vi "RT Driver_Get Date And Time NTP V4.vi"(8 "error in (no error) 2":errorcluster, 10 "port or service name":u16=123, 11 "Timer Server IP Address":string="206.246.122.250") -> (0 "error out":errorcluster, 1 "Last error":errorcluster, 2 "Server Reached":bool, 3 "Server Time (Transmit TimeStamp)":timestamp format="%<%.6X\n%x>T", 5 "Offset (s)":dbl format="%_4p")   [LabVIEW 2013, in "SNTP Light Custom Device Engine.lvlib"]
uses:
  SNTP Light Custom Device Engine.lvlib
panel:
  out "x+y 2":dbl format="%.6f"
  out "x+y":dbl format="%.6f"
  out "Server Time (Receive TimeStamp)":timestamp format="%<%.6X\n%x>T"
  out "Round Trip Delay (s)":dbl
  out "current time":timestamp format="%<%.6X\n%x>T"
  out "Local Time (Destination TimeStamp)":timestamp format="%<%.6X\n%x>T"
  # "64.90.182.55"
  # "129.6.15.28"
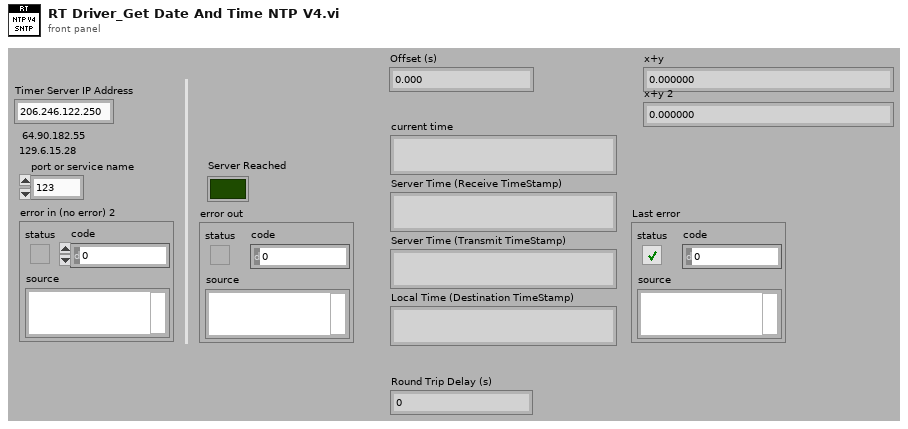
[diagram p1: front panel]
types:
  T1 = cluster{"LI|VN|Mode":u8, "Stratum":u8, "Poll":u8, "Precision":u8, "Root Delay":u32, "Root Dispersion":u32, "Reference Identifier":u32, "Reference Timestamp":fxp<+,64,32>, "Originate Timestamp":fxp<+,64,32>, "Receive Timestamp":fxp<+,64,32>, "Transmit Timestamp":fxp<+,64,32>}
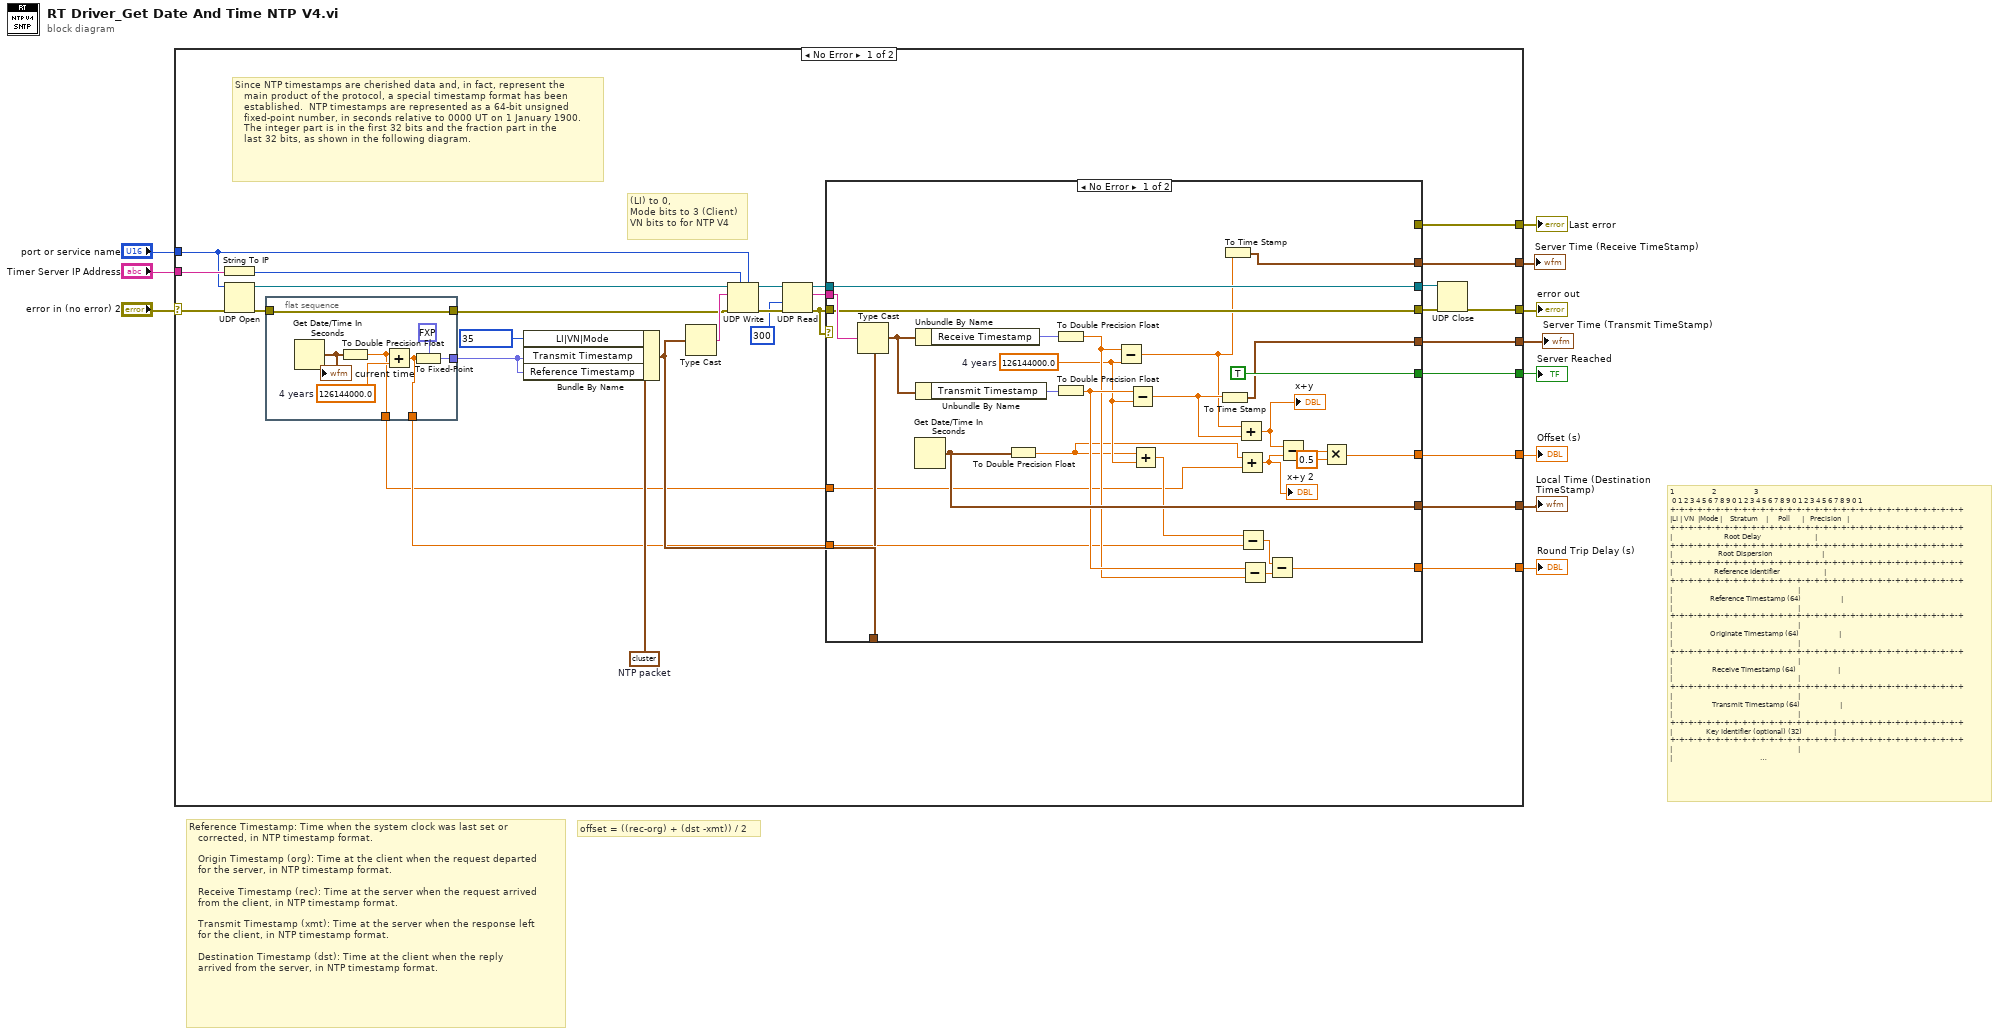
[diagram p0: block diagram]
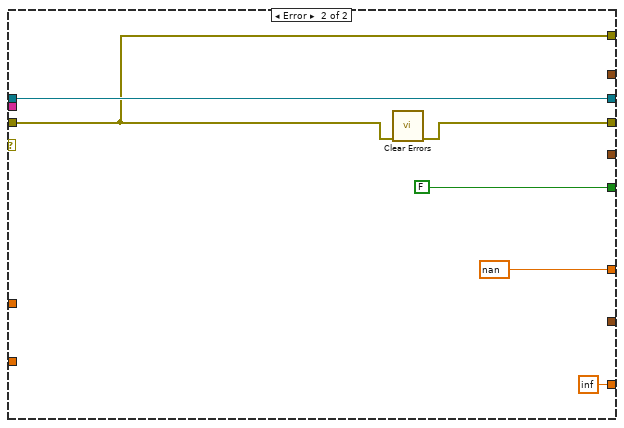
[diagram p2: hidden frame]
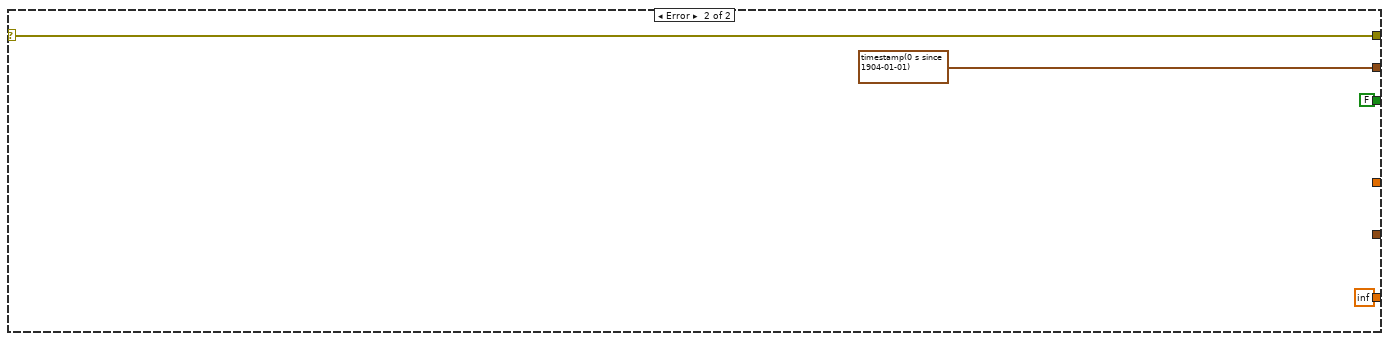
[diagram p3: hidden frame]
diagram:
  # "offset = ((rec-org) + (dst -xmt)) / 2"
  # "Reference Timestamp: Time when the system clock was last set or\n   corrected, in NTP timestamp format.\n\n   Origin Timestamp (org): Time at the client when the request departed\n   for the server, in NTP timestamp format.\n\n   Receive Timestamp (rec): Time at the server when the request arrived\n   from the client, in NTP timestamp format.\n\n   Transmit Timestamp (xmt): Time at the server when the response left\n   for the client, in NTP timestamp format.\n\n   Destination Timestamp (dst): Time at the client when the reply\n   arrived from the server, in NTP timestamp format."
  # "1                   2                   3\n 0 1 2 3 4 5 6 7 8 9 0 1 2 3 4 5 6 7 8 9 0 1 2 3 4 5 6 7 8 9 0 1\n+-+-+-+-+-+-+-+-+-+-+-+-+-+-+-+-+-+-+-+-+-+-+-+-+-+-+-+-+-+-+-+-+\n|LI | VN  |Mode |    Stratum    |     Poll      |   Precision   |\n+-+-+-+-+-+-+-+-+-+-+-+-+-+-+-+-+-+-+-+-+-+-+-+-+-+-+-+-+-+-+-+-+\n|                          Root Delay                           |\n+-+-+-+-+-+-+-+-+-+-+-+-+-+-+-+-+-+-+-+-+-+-+-+-+-+-+-+-+-+-+-+-+\n|                       Root Dispersion                         |\n+-+-+-+-+-+-+-+-+-+-+-+-+-+-+-+-+-+-+-+-+-+-+-+-+-+-+-+-+-+-+-+-+\n|                     Reference Identifier                      |\n+-+-+-+-+-+-+-+-+-+-+-+-+-+-+-+-+-+-+-+-+-+-+-+-+-+-+-+-+-+-+-+-+\n|                                                               |\n|                   Reference Timestamp (64)                    |\n|                                                               |\n+-+-+-+-+-+-+-+-+-+-+-+-+-+-+-+-+-+-+-+-+-+-+-+-+-+-+-+-+-+-+-+-+\n|                                                               |\n|                   Originate Timestamp (64)                    |\n|                                                               |\n+-+-+-+-+-+-+-+-+-+-+-+-+-+-+-+-+-+-+-+-+-+-+-+-+-+-+-+-+-+-+-+-+\n|                                                               |\n|                    Receive Timestamp (64)                     |\n|                                                               |\n+-+-+-+-+-+-+-+-+-+-+-+-+-+-+-+-+-+-+-+-+-+-+-+-+-+-+-+-+-+-+-+-+\n|                                                               |\n|                    Transmit Timestamp (64)                    |\n|                                                               |\n+-+-+-+-+-+-+-+-+-+-+-+-+-+-+-+-+-+-+-+-+-+-+-+-+-+-+-+-+-+-+-+-+\n|                 Key Identifier (optional) (32)                |\n+-+-+-+-+-+-+-+-+-+-+-+-+-+-+-+-+-+-+-+-+-+-+-+-+-+-+-+-+-+-+-+-+\n|                                                               |\n|                                                               |\n|                 Message Digest (optional) (128)               |\n|                                                               |\n|                                                               |\n+-+-+-+-+-+-+-+-+-+-+-+-+-+-+-+-+-+-+-+-+-+-+-+-+-+-+-+-+-+-+-+-+"
  n1 = case shown="No Error" "error in (no error) 2" {
    selector: "error in (no error) 2" -> [w29 w86]
    tunnel: [w39 timestamp(0 s since 1904-01-01)] -> w11
    tunnel: [w24 w86] -> w10
    tunnel: "Timer Server IP Address" -> [w36 _]
    tunnel: [w23 FALSE] -> w7
    tunnel: [w20 _] -> w6
    tunnel: [w18 _] -> w5
    tunnel: "port or service name" -> [w15 _]
    tunnel: [w17 _] -> w3
    tunnel: [w16 inf] -> w2
    tunnel: [w13 _] -> w1
    frame No Error {
      w40 = T1 {"LI|VN|Mode"=0, "Stratum"=0, "Poll"=0, "Precision"=0, "Root Delay"=0, "Root Dispersion"=0, "Reference Identifier"=0, "Reference Timestamp"=0.0, "Originate Timestamp"=0.0, "Receive Timestamp"=0.0, "Transmit Timestamp"=0.0}  # NTP packet
      # "Since NTP timestamps are cherished data and, in fact, represent the\n   main product of the protocol, a special timestamp format has been\n   established.  NTP timestamps are represented as a 64-bit unsigned\n   fixed-point number, in seconds relative to 0000 UT on 1 January 1900.\n   The integer part is in the first 32 bits and the fraction part in the\n   last 32 bits, as shown in the following diagram."
      # "(LI) to 0,\nMode bits to 3 (Client)\nVN bits to for NTP V4"
      n2 = String To IP(1:w36) -> (0:w34:u32)
      n3 = UDP Open(8:w29, 11:w15) -> (port=w33:refnum<k16>, 0:w28:errorcluster)  [unwired: 3 in, 1 out]
      n4 = flat-sequence {
        tunnel: w28 -> [w82]
        tunnel: [w82] -> w14
        tunnel: [w81] -> w21
        tunnel: [w77] -> w19
        tunnel: [w76] -> w12
        frame #0 {
          w78 = 126144000.0  # 4 years
          n5 = Get Date/Time In Seconds() -> (seconds since 1Jan1904=w79:timestamp)
          "current time" <- w79
          n6 = To Double Precision Float(number=w79) -> (double precision float=w76:dbl)
          n7 = Add(x=w76, y=w78) -> (x+y=w77:dbl)
          n8 = To Fixed-Point(fixed-point type=fxp<+,64,32> 0.0 ("Transmit Timestamp"), number=w77) -> (fixed-point=w81:fxp<+,64,32>)
        }
      }
      n9 = Bundle By Name(cluster=w40, "LI|VN|Mode"=u8 35, "Transmit Timestamp"=w21, "Reference Timestamp"=w21) -> (w22:T1)
      n10 = Type Cast(x=w22) -> (*(type *) &x=w37:string)  [unwired: 1 in]
      n11 = UDP Write(address=w34, port or service name=w15, connection ID=w33, data in=w37, 8:w14) -> (error out=w35:errorcluster, 3:w32:refnum<k16>)  [unwired: 1 in]
      n12 = UDP Read(connection ID=w32, timeout ms (25000)=300, 8:w35) -> (data out=w38:string, error out=w27:errorcluster, 3:w31:refnum<k16>)  [unwired: 1 in, 2 out]
      n13 = case shown="No Error" w27 {
        tunnel: w22 -> [w69 _]
        tunnel: [w58 _] -> w39
        tunnel: w38 -> [w67 _]
        tunnel: [w66 w74] -> w25
        tunnel: w31 -> [w65 w75]
        tunnel: w27 -> [w66 w71]
        tunnel: [w65 w75] -> w26
        tunnel: [TRUE FALSE] -> w23
        tunnel: [w44 nan] -> w20
        tunnel: w19 -> [w42 _]
        tunnel: [w57 _] -> w18
        tunnel: [_ w71] -> w17
        tunnel: [w52 inf] -> w16
        tunnel: [w49 _] -> w13
        tunnel: w12 -> [w43 _]
        frame No Error {
          w50 = 126144000.0  # 4 years
          n14 = Type Cast(type=w69, x=w67) -> (*(type *) &x=w63:T1)
          n15 = Get Date/Time In Seconds() -> (seconds since 1Jan1904=w57:timestamp)
          n16 = Unbundle By Name(w63) -> ("Receive Timestamp"=w68:fxp<+,64,32>)
          n17 = Unbundle By Name(w63) -> ("Transmit Timestamp"=w62:fxp<+,64,32>)
          n18 = To Double Precision Float(number=w57) -> (double precision float=w45:dbl)
          n19 = To Double Precision Float(number=w68) -> (double precision float=w51:dbl)
          n20 = To Double Precision Float(number=w62) -> (double precision float=w53:dbl)
          n21 = Subtract(x=w51, y=w50) -> (x-y=w46:dbl)
          n22 = Subtract(x=w53, y=w50) -> (x-y=w47:dbl)
          n23 = Add(x=w45, y=w50) -> (x+y=w56:dbl)
          n24 = To Time Stamp(1:w47) -> (0:w58:timestamp)
          n25 = To Time Stamp(1:w46) -> (0:w49:timestamp)
          n26 = Add(x=w46, y=w47) -> (x+y=w61:dbl)
          "x+y" <- w61
          n27 = Add(x=w45, y=w43) -> (x+y=w48:dbl)
          "x+y 2" <- w48
          n28 = Subtract(x=w56, y=w42) -> (x-y=w55:dbl)
          n29 = Subtract(x=w53, y=w51) -> (x-y=w54:dbl)
          n30 = Subtract(x=w55, y=w54) -> (x-y=w52:dbl)
          n31 = Subtract(x=w61, y=w48) -> (x-y=w60:dbl)
          n32 = Multiply(x=w60, y=0.5) -> (x*y=w44:dbl)
        }
        frame Error {
          n33 = call <vilib>:"Clear Errors.vi"("error in (no error)"=w71) -> ("error out"=w74:errorcluster)  [unwired: 6 in]
        }
      }
      n34 = UDP Close(connection ID=w26, 8:w25) -> (error out=w24:errorcluster)  [unwired: 1 out]
    }
    frame Error {
    }
  }
  "Server Time (Transmit TimeStamp)" <- w11
  "error out" <- w10
  "Server Reached" <- w7
  "Offset (s)" <- w6
  "Local Time (Destination TimeStamp)" <- w5
  "Last error" <- w3
  "Round Trip Delay (s)" <- w2
  "Server Time (Receive TimeStamp)" <- w1
